vi "Delete.vi"(8 "error in (no error)":errorcluster, 11 "MatchData in":refnum<class "MatchData.lvclass">) -> (0 "error out":errorcluster, 3 "MatchData out":refnum<class "MatchData.lvclass">)   [LabVIEW 2019, in "MatchData.lvclass"]
uses:
  MatchData.lvclass
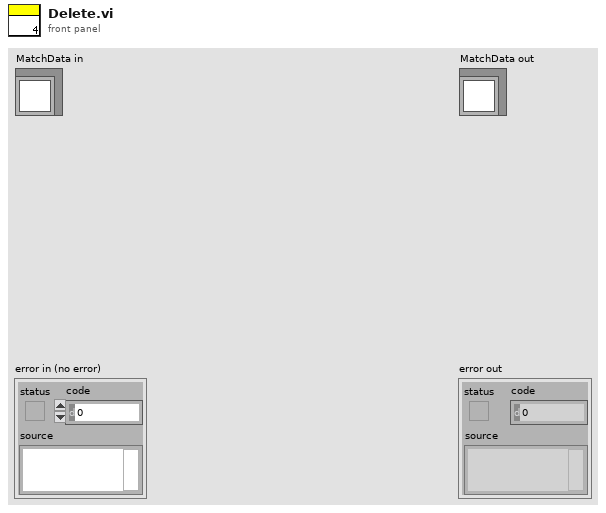
[diagram p1: front panel]
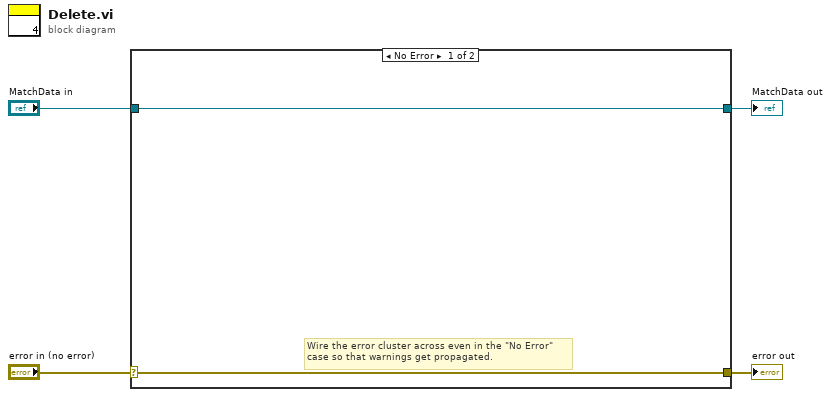
[diagram p0: block diagram]
diagram:
  n1 = case shown="No Error" "error in (no error)" {
    selector: "error in (no error)" -> [w5 w8]
    tunnel: [w5 w8] -> w3
    tunnel: [w6 w7] -> w1
    tunnel: "MatchData in" -> [w6 w7]
    frame No Error {
      # "Wire the error cluster across even in the \"No Error\"\ncase so that warnings get propagated."
    }
    frame Error {
    }
  }
  "error out" <- w3
  "MatchData out" <- w1
